vi "SerialTorqueCalibration.vi"() -> ()   [LabVIEW 2017]
uses:
  <vilib>/Analysis/baseanly.llb/Mean (DBL).vi
  <vilib>/Instr/_visa.llb/VISA Configure Serial Port (Instr).vi
  <vilib>/express/express shared/transition.llb/Dynamic To Waveform Array.vi
  <vilib>/express/express signal manip/GetorSetDDTAttributes/Set DDT Attributes/SetT0.vi
  <vilib>/express/express shared/transition.llb/Waveform Array To Dynamic.vi
  <vilib>/express/express signal manip/GetorSetDDTAttributes/Set DDT Attributes/Set DDT Properties.xnode
  <vilib>/Analysis/NI_AALBase.lvlib
  <vilib>/Analysis/NI_AALPro.lvlib
panel:
  out "Quadratic Coefficients":dbl[](array[numeric])
  out "Linear Coefficients":dbl[](array[numeric])
  in  "Filename":path=path "test.tdms"
  in  "Save Data":bool
  in  "Baud Rate":dbl=115200.0
  in  "Moment Arm Units":u16(ring) items=["in", "cm"]
  in  "Weight Units":u16(ring) items=["lb", "kg", "oz"]
  out "Torque Array (kg-cm)":dbl[](array[numeric])
  out "ADC Value Array":dbl[](array[numeric])
  out "ADC Value vs Troque":cluster{dbl[], dbl[]}(graph)
  out "Average ADC Value":dbl format="%0.2f"
  out "Live ADC Value":cluster{i32, dbl, dbl[]}(graph)
  in  "Com Port":refnum<visa-resource-name>="ASRL1::INSTR"
  in  "Sample Frequency":dbl=200.0
  in  "Number of Samples":dbl=100.0
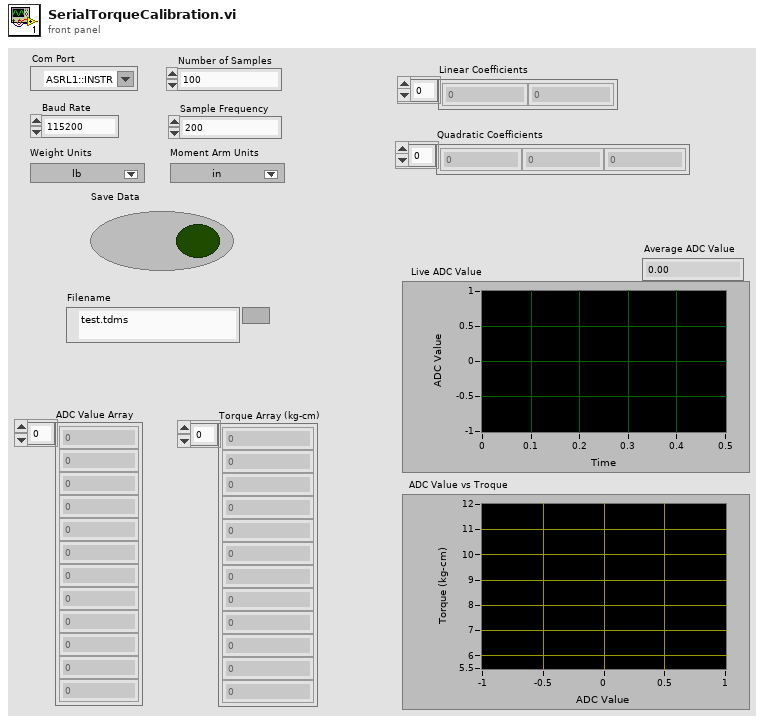
[diagram p1: front panel]
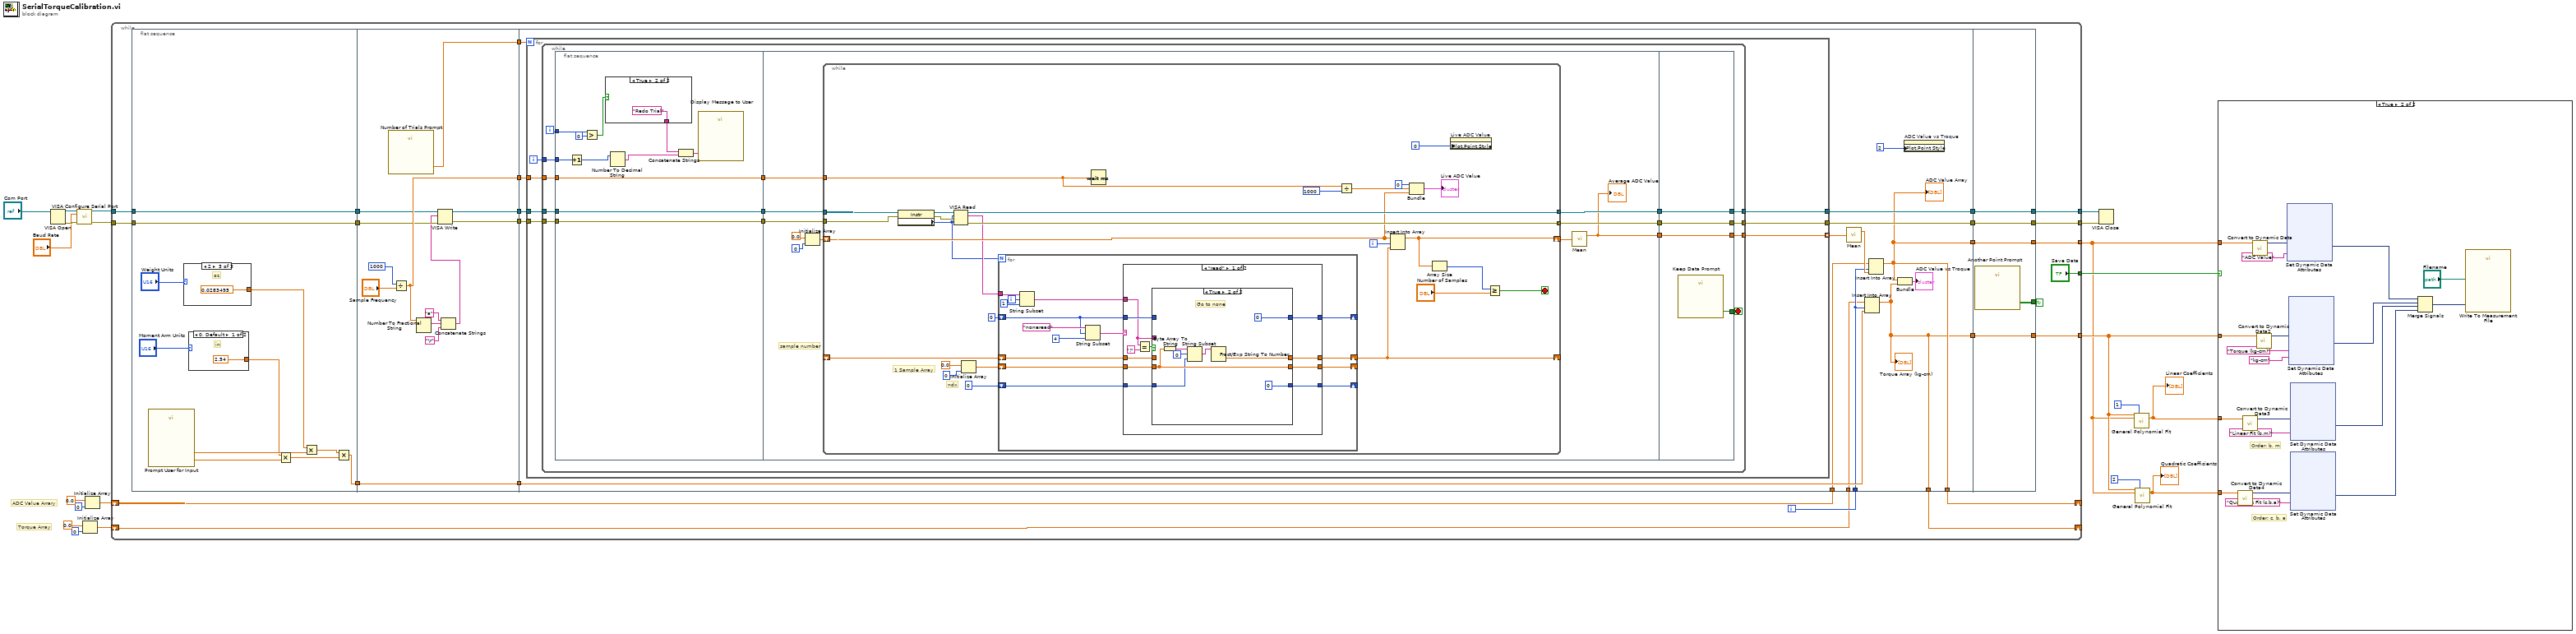
[diagram p0: block diagram]
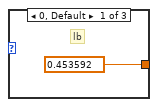
[diagram p3: hidden frame]
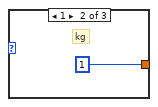
[diagram p4: hidden frame]
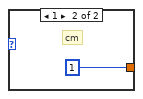
[diagram p5: hidden frame]
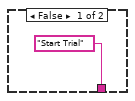
[diagram p6: hidden frame]
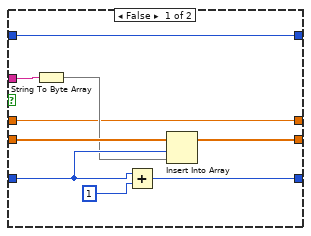
[diagram p7: hidden frame]
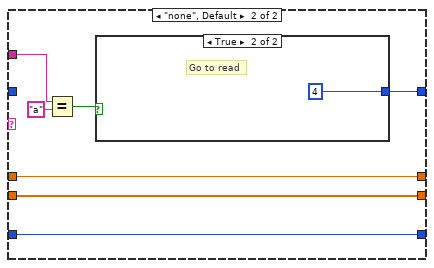
[diagram p8: hidden frame]
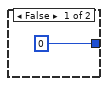
[diagram p9: hidden frame]
diagram:
  # "Torque Array"
  # "ADC Value Arrary"
  n1 = VISA Open(VISA resource name="Com Port") -> (VISA resource name=w20:refnum<visa-resource-name>, error out=w19:errorcluster)  [unwired: 4 in]
  n2 = call-poly "VISA Configure Serial Port"("VISA resource name"=w20, "baud rate (9600)"="Baud Rate", "error in (no error)"=w19) -> ("VISA resource name out"=w18:refnum<visa-resource-name>, "error out"=w17:errorcluster)  [unwired: 11 in]
  n3 = Initialize Array(0.0 ("element"), 0 ("dimension size")) -> (w9:dbl[])
  n4 = Initialize Array(0.0 ("element"), 0 ("dimension size")) -> (w10:dbl[])
  n5 = while {
    tunnel: w18 -> [w44]
    tunnel: w17 -> [w43]
    tunnel: [w40] -> w16
    tunnel: [w39] -> w15
    shift-right: [w29] -> _
    shift-left: w10 -> [w31]
    shift-right: [w28] -> _
    shift-left: w9 -> [w30]
    tunnel: ["Save Data"] -> w7
    tunnel: [w24] -> w3
    tunnel: [w22] -> w4
    i -> [w32]
    stop <- w46 continue-if-true
    n6 = flat-sequence {
      tunnel: w43 -> [w56]
      tunnel: w44 -> [w57]
      tunnel: [w57] -> w36
      tunnel: [w56] -> w35
      tunnel: [w55] -> w33
      tunnel: [w75] -> w45
      tunnel: [w64] -> w42
      tunnel: [w71] -> w37
      tunnel: w36 -> [w67]
      tunnel: w35 -> [w66]
      tunnel: [w72] -> w34
      tunnel: w33 -> [w72]
      tunnel: [w65] -> w27
      tunnel: w45 -> [w91]
      tunnel: w42 -> [w89]
      tunnel: [w88] -> w41
      tunnel: [w87] -> w38
      tunnel: w37 -> [w86]
      tunnel: w34 -> [w84]
      tunnel: w32 -> [w82]
      tunnel: w31 -> [w81]
      tunnel: w30 -> [w80]
      tunnel: [w78] -> w29
      tunnel: [w77] -> w28
      tunnel: w27 -> [w90]
      tunnel: [w78] -> w25
      tunnel: [w77] -> w23
      tunnel: [w224] -> w46
      tunnel: w41 -> [w223]
      tunnel: [w223] -> w40
      tunnel: [w222] -> w39
      tunnel: w38 -> [w222]
      tunnel: w25 -> [w221]
      tunnel: [w221] -> w24
      tunnel: w23 -> [w220]
      tunnel: [w220] -> w22
      frame #0 {
        n7 = call "Prompt User for Input"() -> ("Moment Arm"=w48:dbl, "Weight"=w51:dbl)  [unwired: 16 in, 2 out]
        n8 = case shown="2" "Weight Units" {
          tunnel: [0.453592 1 0.0283495] -> w52
          frame 0, Default {
            # "lb"
          }
          frame 1 {
            # "kg"
          }
          frame 2 {
            # "oz"
          }
        }
        n9 = case shown="0, Default" "Moment Arm Units" {
          tunnel: [2.54 1] -> w47
          frame 0, Default {
            # "in"
          }
          frame 1 {
            # "cm"
          }
        }
        n10 = Multiply(x=w47, y=w48) -> (x*y=w49:dbl)
        n11 = Multiply(x=w52, y=w51) -> (x*y=w50:dbl)
        n12 = Multiply(x=w50, y=w49) -> (x*y=w55:dbl)
      }
      frame #1 {
        n13 = call "Number of Trials Prompt"() -> ("Trails"=w75:dbl)  [unwired: 17 in, 2 out]
        n14 = Divide(x=1000, y="Sample Frequency") -> (x/y=w71:dbl)
        n15 = Number To Fractional String(number=w71) -> (F-format string=w69:string)  [unwired: 3 in]
        n16 = Concatenate Strings("a", w69, "\r") -> (w63:string)
        n17 = VISA Write(VISA resource name=w67, write buffer=w63, error in (no error)=w66) -> (VISA resource name out=w65:refnum<visa-resource-name>, error out=w64:errorcluster)  [unwired: 1 out]
      }
      frame #2 {
        n18 = for {
          N: w91 -> [_]
          tunnel: w90 -> [w98]
          tunnel: w89 -> [w97]
          tunnel: [w96] -> w88
          tunnel: [w95] -> w87
          tunnel: w86 -> [w94]
          tunnel: [w93] -> w85 mode=indexing
          i -> [w92]
          n19 = while {
            tunnel: w98 -> [w112]
            tunnel: w97 -> [w111]
            tunnel: [w109] -> w96
            tunnel: [w108] -> w95
            tunnel: w94 -> [w106]
            tunnel: [w104] -> w93
            tunnel: w92 -> [w99]
            i -> [w100]
            stop <- w113 stop-if-true
            n20 = flat-sequence {
              tunnel: w106 -> [w122]
              tunnel: w111 -> [w123]
              tunnel: w112 -> [w124]
              tunnel: [w124] -> w103
              tunnel: [w123] -> w102
              tunnel: [w122] -> w101
              tunnel: w100 -> [w119]
              tunnel: w99 -> [w116]
              tunnel: [w134] -> w110
              tunnel: [w133] -> w107
              tunnel: [w127] -> w105
              tunnel: w103 -> [w136]
              tunnel: w102 -> [w135]
              tunnel: w101 -> [w132]
              tunnel: [w219] -> w113
              tunnel: w110 -> [w218]
              tunnel: [w218] -> w109
              tunnel: [w217] -> w108
              tunnel: w107 -> [w217]
              tunnel: w105 -> [w216]
              tunnel: [w216] -> w104
              frame #0 {
                n21 = Increment(x=w116) -> (x+1=w115:i32)
                n22 = Greater?(x=w119, y=0) -> (0:w118:bool)
                n23 = case shown="True" w118 {
                  tunnel: ["Start Trial" "Redo Trial"] -> w117
                  frame False {
                  }
                  frame True {
                  }
                }
                n24 = Number To Decimal String(number=w115) -> (decimal integer string=w114:string)  [unwired: 1 in]
                n25 = Concatenate Strings(w117, w114) -> (w121:string)
                n26 = call "Display Message to User"("Message"=w121) -> ()  [unwired: 9 in, 2 out]
              }
              frame #1 {
                # "sample number"
                n27 = Initialize Array(0.0, 0 ("dimension size")) -> (w131:dbl[])
                n28 = while {
                  tunnel: w136 -> [w161]
                  tunnel: w135 -> [w160]
                  tunnel: [w159] -> w134
                  tunnel: [w158] -> w133
                  shift-right: [w146] -> _
                  shift-left: _ -> [w152]
                  tunnel: w132 -> [w141]
                  shift-right: [w144] -> w128
                  shift-left: w131 -> [w145]
                  i -> [w147]
                  stop <- w150 stop-if-true
                  # "ndx"
                  # "1 Sample Array"
                  n29 = property class="Instr"(reference=w161, error in=w160) -> (reference out=w163:refnum<visa-resource-name>, error out=w162:errorcluster, "Serial Settings:Number of Bytes at Serial Port"=w138:u32)
                  n30 = VISA Read(VISA resource name=w163, byte count=w138, error in (no error)=w162) -> (VISA resource name out=w159:refnum<visa-resource-name>, read buffer=w139:string, error out=w158:errorcluster)  [unwired: 1 out]
                  n31 = Initialize Array(0.0 ("element"), 0 ("dimension size")) -> (w154:dbl[])
                  n32 = for {
                    N: w138 -> [_]
                    tunnel: w139 -> [w177]
                    shift-right: [w173] -> _
                    shift-left: 0 -> [w172]
                    shift-right: [w168] -> _
                    shift-left: w154 -> [w169]
                    shift-right: [w167] -> _
                    shift-left: 0 ("dimension size") -> [w170]
                    shift-right: [w166] -> w146
                    shift-left: w152 -> [w165]
                    i -> [w176]
                    n33 = String Subset(string=w177, offset (0)=w176, length (rest)=1 ("length (rest)")) -> (substring=w171:string)
                    n34 = String Subset(string="noneread", offset (0)=w172, length (rest)=4 ("length (rest)")) -> (substring=w164:string)
                    n35 = case shown="\"read\"" w164 {
                      tunnel: [w189 w211] -> w173
                      tunnel: w172 -> [w188 _]
                      tunnel: w171 -> [w185 w210]
                      tunnel: w170 -> [w184 w207]
                      tunnel: w169 -> [w183 w208]
                      tunnel: [w182 w208] -> w168
                      tunnel: [w181 w207] -> w167
                      tunnel: [w180 w209] -> w166
                      tunnel: w165 -> [w179 w209]
                      frame "read" {
                        n36 = Equal?(x=w185, y="!") -> (x = y?=w187:bool)
                        n37 = case shown="True" w187 {
                          tunnel: [w198 0] -> w189
                          tunnel: w188 -> [w198 _]
                          tunnel: w185 -> [w195 _]
                          tunnel: w184 -> [w196 w200]
                          tunnel: w183 -> [w197 w203]
                          tunnel: [w193 w203] -> w182
                          tunnel: [w192 0] -> w181
                          tunnel: [w191 w205] -> w180
                          tunnel: w179 -> [w191 _]
                          frame False {
                            n38 = String To Byte Array(string=w195) -> (unsigned byte array=w194:u8[])
                            n39 = Add(x=w196, y=1 ("dimension size")) -> (x+y=w192:i32)
                            n40 = Insert Into Array(array=w197, index=w196, new element=w194) -> (w193:dbl[])
                          }
                          frame True {
                            # "Go to none"
                            n41 = Byte Array To String(unsigned byte array=w203) -> (string=w202:string)
                            n42 = String Subset(string=w202, offset (0)=0, length (rest)=w200) -> (substring=w201:string)
                            n43 = Fract/Exp String To Number(string=w201) -> (number=w205:dbl)  [unwired: 3 in, 1 out]
                          }
                        }
                      }
                      frame "none", Default {
                        n44 = Equal?(x=w210, y="a") -> (x = y?=w213:bool)
                        n45 = case shown="True" w213 {
                          tunnel: [0 4] -> w211
                          frame False {
                          }
                          frame True {
                            # "Go to read"
                          }
                        }
                      }
                    }
                  }
                  n46 = Wait (ms)(milliseconds to wait=w141) -> ()  [unwired: 1 out]
                  n47 = Divide(x=w141, y=1000) -> (x/y=w140:dbl)
                  n48 = Insert Into Array(array=w145, index=w147, new element=w146) -> (w144:dbl[])
                  n49 = Bundle(0, w140, w145) -> (→"Live ADC Value":cluster{i32, dbl, dbl[]})  [unwired: 1 in]
                  n50 = Array Size(array=w144) -> (size(s)=w143:i32)
                  n51 = property on="Live ADC Value" class="WFGraph (strict)"("Plot.Point Style"=u8 0) -> ()  [unwired: 2 in, 2 out]
                  n52 = Greater Or Equal?(x=w143, y="Number of Samples") -> (x >= y?=w150:bool)
                }
                n53 = call-poly <vilib>:"Mean.vi"("X"=w128) -> ("mean"=w127:dbl)  [unwired: 1 out]
                "Average ADC Value" <- w127
              }
              frame #2 {
                n54 = call "Keep Data Prompt"() -> ("OK"=w219:bool)  [unwired: 18 in, 1 out]
              }
            }
          }
        }
        n55 = call-poly <vilib>:"Mean.vi"("X"=w85) -> ("mean"=w83:dbl)  [unwired: 1 out]
        n56 = Insert Into Array(array=w80, index=w82, new element=w84) -> (w77:dbl[])
        "Torque Array (kg-cm)" <- w77
        n57 = Insert Into Array(array=w81, index=w82, new element=w83) -> (w78:dbl[])
        "ADC Value Array" <- w78
        n58 = Bundle(w78, w77) -> (→"ADC Value vs Troque":cluster{dbl[], dbl[]})  [unwired: 1 in]
        n59 = property on="ADC Value vs Troque" class="XYGraph (strict)"("Plot.Point Style"=u8 2) -> ()  [unwired: 2 in, 2 out]
      }
      frame #3 {
        n60 = call "Another Point Prompt"() -> ("OK"=w224:bool)  [unwired: 18 in, 1 out]
      }
    }
  }
  n61 = VISA Close(VISA resource name=w16, error in (no error)=w15) -> ()  [unwired: 1 out]
  n62 = call <vilib>:"General Polynomial Fit.vi"("Y"=w4, "polynomial order"=1, "X"=w3) -> ("Polynomial Coefficients"=w2:dbl[])  [unwired: 9 in, 3 out]
  "Linear Coefficients" <- w2
  n63 = call <vilib>:"General Polynomial Fit.vi"("Y"=w4, "polynomial order"=2, "X"=w3) -> ("Polynomial Coefficients"=w1:dbl[])  [unwired: 9 in, 3 out]
  "Quadratic Coefficients" <- w1
  n64 = case shown="True" w7 {
    tunnel: w3 -> [_ w243]
    tunnel: w4 -> [_ w240]
    tunnel: w2 -> [_ w236]
    tunnel: w1 -> [_ w235]
    frame False {
    }
    frame True {
      # "Order: c, b, a"
      # "Order: b, m"
      n65 = call "Convert to Dynamic Data4"("Array"=w235) -> ("Dynamic Data Type"=w233:dynamicdata)  [unwired: 3 in]
      n66 = call "Convert to Dynamic Data3"("Array"=w236) -> ("Dynamic Data Type"=w234:dynamicdata)  [unwired: 3 in]
      n67 = call "Convert to Dynamic Data"("Array"=w243) -> ("Dynamic Data Type"=w242:dynamicdata)  [unwired: 3 in]
      n68 = call "Convert to Dynamic Data2"("Array"=w240) -> ("Dynamic Data Type"=w239:dynamicdata)  [unwired: 3 in]
      n69 = xnode "Set Dynamic Data Attributes"("Signals In"=w242, "Signal Name"="ADC Value") -> ("Signals Out"=w230:dynamicdata)  [unwired: 2 in, 1 out]
      n70 = xnode "Set Dynamic Data Attributes"("Signals In"=w239, "Signal Name"="Torque (kg-cm)", "Unit"="kg-cm") -> ("Signals Out"=w229:dynamicdata)  [unwired: 2 in, 1 out]
      n71 = xnode "Set Dynamic Data Attributes"("Signals In"=w234, "Signal Name"="Linear Fit (b,m)") -> ("Signals Out"=w228:dynamicdata)  [unwired: 2 in, 1 out]
      n72 = xnode "Set Dynamic Data Attributes"("Signals In"=w233, "Signal Name"="Quadratic Fit (c,b,a)") -> ("Signals Out"=w227:dynamicdata)  [unwired: 2 in, 1 out]
      n73 = Merge Signals(w230, w229, w228, w227) -> (w226:dynamicdata)
      n74 = call "Write To Measurement File"("Signals"=w226, "Filename"="Filename") -> ()  [unwired: 15 in, 3 out]
    }
  }
